vi "XY Graph Clear Event.vi"(8 "Error In":errorcluster, 11 "XYGraph Ref":T1) -> (0 "Error Out":errorcluster, 1 "Message":string, 3 "Graph Caption (or Label)":string)   [LabVIEW 2021, in "XY Graph Add-Ons.lvlib"]
uses:
  XY Graph Add-Ons.lvlib
  XY Graph Refnum.ctl
  Arrays/Arrays.lvlib
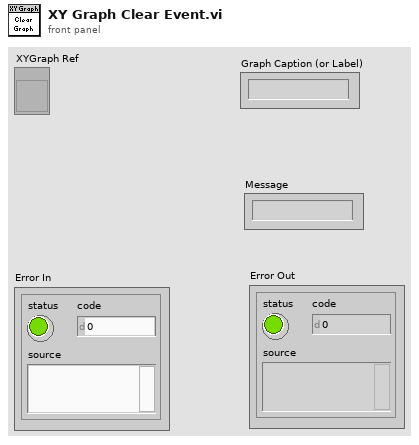
[diagram p1: front panel]
types:
  T1 = typedef "XY Graph Add-Ons.lvlib/XY Graph Refnum.ctl" = refnum<vi>
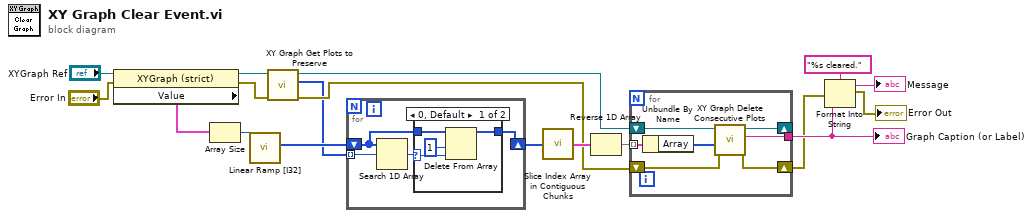
[diagram p0: block diagram]
diagram:
  n1 = property class="XYGraph (strict)"(reference="XYGraph Ref", error in="Error In") -> (reference out=w10:T1, error out=w8:errorcluster, "Value"=w11:cluster{"X Array":dbl[], "Y Array":dbl[]}[])
  n2 = Array Size(array=w11) -> (size(s)=w13:i32)
  n3 = call "Linear Ramp [I32].vi"("# Elements"=w13) -> ("Ramp"=w12:i32[])  [unwired: 8 in]
  n4 = call "XY Graph Get Plots to Preserve.vi"("Error In"=w8, "XYGraph in"=w10) -> ("Error Out"=w7:errorcluster, "Preserved Plots"=w6:i32[], "XYGraph dup"=w9:T1)  [unwired: 6 in, 1 out]
  n5 = for {
    tunnel: w6 -> [w22] mode=indexing
    shift-right: [w19] -> w18
    shift-left: w12 -> [w20]
    n6 = Search 1D Array(1D array=w20, element=w22) -> (index of element=w21:i32)  [unwired: 1 in]
    n7 = case shown="0, Default" w21 {
      selector: w21 -> [w25 _]
      tunnel: w20 -> [w26 w27]
      tunnel: [w24 w27] -> w19
      frame 0, Default {
        n8 = Delete From Array(array=w26, length=1, index=w25) -> (array with subset deleted=w24:i32[])  [unwired: 1 out]
      }
      frame -1 {
      }
    }
  }
  n9 = call "Slice Index Array in Contiguous Chunks.vi"("Array in"=w18) -> ("Contiguous sub-Arrays"=w17:cluster{"Array":i32[]}[])  [unwired: 8 in]
  n10 = Reverse 1D Array(array=w17) -> (reversed array=w16:cluster{"Array":i32[]}[])
  n11 = for {
    tunnel: w16 -> [w34] mode=indexing
    shift-right: [w31] -> _
    shift-left: w9 -> [w32]
    tunnel: [w30] -> w5
    shift-right: [w28] -> w2
    shift-left: w7 -> [w29]
    n12 = Unbundle By Name(w34) -> ("Array"=w33:i32[])
    n13 = call "XY Graph Delete Consecutive Plots.vi"("Error In"=w29, "Plot Indices"=w33, "XYGraph Ref"=w32) -> ("Error Out"=w28:errorcluster, "Graph Caption (or Label)"=w30:string, "XYGraph Ref"=w31:refnum<vi>)  [unwired: 5 in, 1 out]
  }
  "Graph Caption (or Label)" <- w5
  n14 = Format Into String(format string="%s cleared.", error in=w2, w5) -> (resulting string=→"Message":string, error out=→"Error Out":errorcluster)  [unwired: 1 in]
